vi "Stop Core.vi"(10 "final error code":i32, 11 "Bioreactor in":refnum<class "Bioreactor.lvclass">) -> (3 "Bioreactor out":refnum<class "Bioreactor.lvclass">)   [LabVIEW 2012, in "Bioreactor Actor.lvlib" / "Bioreactor.lvclass"]
uses:
  Bioreactor.lvclass
  Bioreactor.lvclass/Bioreactor.ctl
  <vilib>/ActorFramework/Actor/Actor.lvclass
  Read VISA resource name.vi
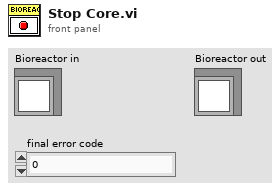
[diagram p1: front panel]
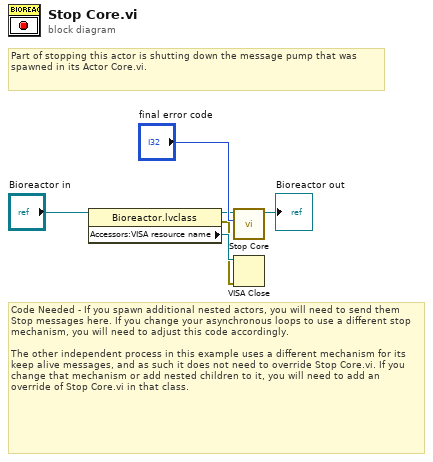
[diagram p0: block diagram]
diagram:
  # "Code Needed - If you spawn additional nested actors, you will need to send them Stop messages here. If you change your asynchronous loops to use a different stop mechanism, you will need to adjust this code accordingly.\n\nThe other independent process in this example uses a different mechanism for its keep alive messages, and as such it does not need to override Stop Core.vi. If you change that mechanism or add nested children to it, you will need to add an override of Stop Core.vi in that class."
  # "Part of stopping this actor is shutting down the message pump that was spawned in its Actor Core.vi."
  n1 = property class="Bioreactor.lvclass"(reference="Bioreactor in") -> (reference out=w3:refnum<class "Bioreactor.lvclass">, error out=w1:errorcluster, "Accessors:VISA resource name"=w2:refnum<visa-resource-name>)  [unwired: 1 in]
  n2 = call-parent "Stop Core.vi"("final error code"="final error code", "Actor in"=w3) -> ("Actor out"=→"Bioreactor out":refnum<class "Bioreactor.lvclass">)  [unwired: 9 in]
  n3 = VISA Close(VISA resource name=w2, error in (no error)=w1) -> ()  [unwired: 1 out]
